vi "Actor Core.vi"(8 "error in":errorcluster, 11 "Communication Clients in":refnum<class "Communication Clients.lvclass">) -> (0 "error out":errorcluster, 3 "Actor out":refnum<class "Actor.lvclass">)   [LabVIEW 2017]
doc: "(<B>Filename</B>: Actor Framework.lvlib:Actor.lvclass:Actor Core.vi)\n\nReceives messages to the actor, reacts to them, and initiates any error handling that may shut the actor down.\n\nDescendant classes may override this VI to append parallel tasks for the actor to complete while it handles messages. Overrides use the Call Parent Method node."
uses:
  Communication Clients.lvclass
  C:/Program Files (x86)/National Instruments/LabVIEW 2017/vi.lib/ActorFramework/Actor/Actor.lvclass
  <vilib>/ActorFramework/Actor/Actor.lvclass
panel:
  out "System String Array":string[](array[string])
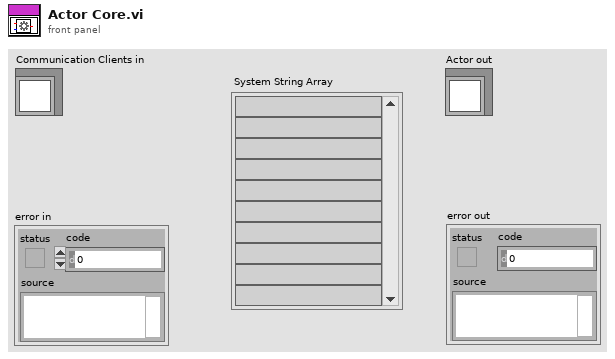
[diagram p1: front panel]
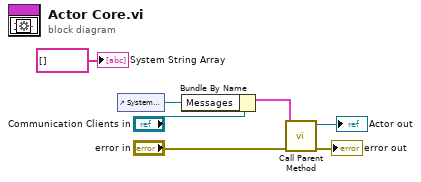
[diagram p0: block diagram]
diagram:
  n1 = control-ref of="System String Array"() -> (w2:refnum<vi>)
  n2 = Bundle By Name(cluster="Communication Clients in", "Messages"=w2) -> (w3:cluster{})
  n3 = call-parent "Call Parent Method"("error in"="error in", "Actor in"=w3) -> ("error out"=→"error out":errorcluster, "Actor out"=→"Actor out":refnum<class "Actor.lvclass">)  [unwired: 8 in]
  "System String Array" <- string[] [] ("System String Array")
